vi "Global_pixelvalue.vi"() -> ()   [LabVIEW 2020]
panel:
  in  "Array - Numeric":dbl[](array[numeric])
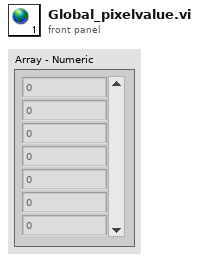
[diagram p1: front panel]
diagram:
